vi "Clear Table.vi"(8 "error in":errorcluster, 11 "Table in":refnum<vi>) -> (0 "error out":errorcluster)   [LabVIEW 2025, in "CAN-LIN Raw Bus Capture UI.lvlib"]
uses:
  CAN-LIN Raw Bus Capture UI.lvlib
  <vilib>/Utility/miscctls.llb/LVRowAndColumnTypeDef.ctl
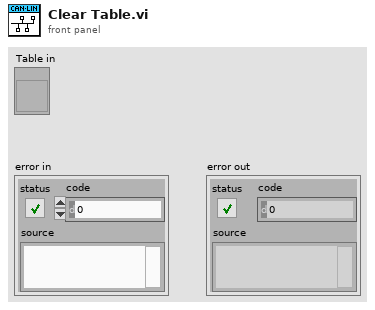
[diagram p1: front panel]
types:
  T1 = typedef "LVRowAndColumnTypeDef.ctl" = cluster{"Row":i32, "Column":i32}
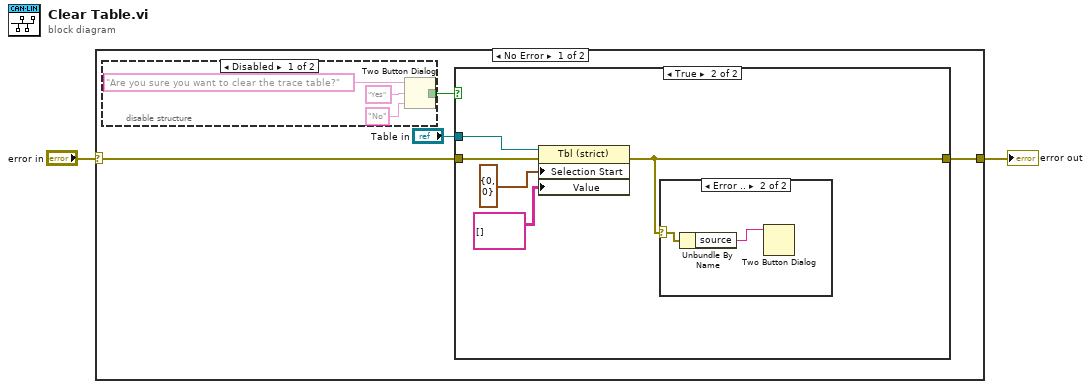
[diagram p0: block diagram]
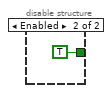
[diagram p2: hidden frame]
diagram:
  n1 = case shown="No Error" "error in" {
    selector: "error in" -> [w3 w20]
    tunnel: [w4 w20] -> w1
    frame No Error {
      n2 = disable-structure shown="Disabled" {
        disable-tunnel: [w7 TRUE ("T button?")] -> w5
        frame Disabled {
          n3 = Two Button Dialog(message="Are you sure you want to clear the trace table?", 1:"No" ("F button name (\"Cancel\")"), 2:"Yes" ("T button name (\"OK\")")) -> (T button?=w7:bool)
        }
        frame Enabled {
        }
      }
      n4 = case shown="True" w5 {
        tunnel: "Table in" -> [_ w17]
        tunnel: [w12 w13] -> w4
        tunnel: w3 -> [w12 w14]
        frame False {
        }
        frame True {
          n5 = property class="Tbl (strict)"(reference=w17, error in=w14, "Selection Start"=T1 {"Row"=0, "Column"=0}, "Value"=string[][] [] ("Captured Data")) -> (error out=w13:errorcluster)  [unwired: 1 out]
          n6 = case shown="Error .." w13 {
            selector: w13 -> [_ w19]
            frame No Error {
            }
            frame Error {
              n7 = Unbundle By Name(w19) -> ("source"=w18:string)
              n8 = Two Button Dialog(message=w18) -> ()  [unwired: 2 in, 1 out]
            }
          }
        }
      }
    }
    frame Error {
    }
  }
  "error out" <- w1
